vi "CheckIfLibraryBannerDefault.vi"(11 "Icon":refnum<class "Icon.lvclass">) -> (2 "DefaultIcon":bool, 3 "Icon out":refnum<class "Icon.lvclass">)   [LabVIEW 2014, in "ClassIconTools.lvlib"]
uses:
  ClassIconTools.lvlib
  <vilib>/LabVIEW Icon API/lv_icon/Classes/Icon/Icon.lvclass
  <vilib>/LabVIEW Icon API/LabVIEW Icon API.lvlib
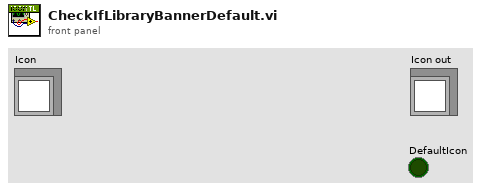
[diagram p1: front panel]
types:
  T1 = typedef "LabVIEW Icon Stored Information.ctl" = cluster{"Text Visible?":bool, "Text Opacity":u8, "Templ Visible?":bool, "Templ Opacity":u8, "Relative Path from 1 to 2":path, "Image":picture, "All User Layers":refnum<class "Layer.lvclass">[], "Body Text":T2}
  T2 = typedef "BodyText.ctl" = cluster{"Line 1 text":string, "Line 2 text":string, "Line 3 text":string, "Line 4 text":string, "Line 1 color":u32, "Line 2 color":u32, "Line 3 color":u32, "Line 4 color":u32, "Body Text Spec":cluster{"Font":T3, "Alignment":T4, "Size":u8}, "Center text vertically":bool, "Capitalize Text":bool}
  T3 = typedef "Font.ctl" = string
  T4 = typedef "Alignment.ctl" = u16
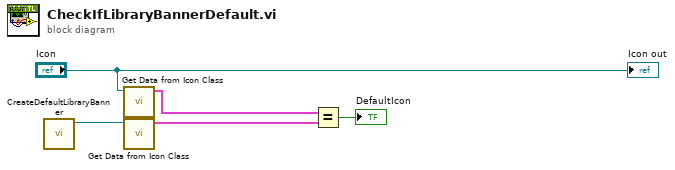
[diagram p0: block diagram]
diagram:
  n1 = call "CreateDefaultLibraryBanner.vi"() -> ("Icon"=w2:refnum<class "Icon.lvclass">)  [unwired: 11 in]
  n2 = call <vilib>:"Get Data from Icon Class.vi"("Icon in"="Icon") -> ("Icon data"=w4:T1)  [unwired: 7 in, 3 out]
  n3 = call <vilib>:"Get Data from Icon Class.vi"("Icon in"=w2) -> ("Icon data"=w3:T1)  [unwired: 7 in, 3 out]
  n4 = Equal?(x=w4, y=w3) -> (x = y?=→"DefaultIcon":bool)
  "Icon out" <- "Icon"
